vi "MachineInfos.vi"() -> ()   [LabVIEW 2013]
panel:
  in  "MachineInfos":T1
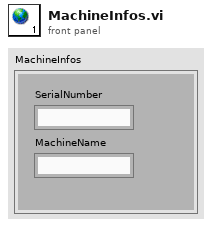
[diagram p1: front panel]
types:
  T1 = cluster{"SerialNumber":string, "MachineName":string}
diagram:
